vi "Write ECAT VARs.vi"(7 "R/W Case":T7, 8 "error in (no error)":errorcluster, 9 "Input FIFO buffer in":dbl[](array[numeric]), 10 "I/O Output Data in":T1 {"BD Refs"."Data Reference" format="%.0x"}, 11 "I/O Imput Vars in":T4[](array[typedef]) {"VS ref" format="%.0x"}) -> (0 "error out":errorcluster, 1 "Input FIFO buffer out":dbl[](array[numeric]), 2 "I/O Output Data out":T1 {"BD Refs"."Data Reference" format="%.0x"}, 3 "I/O Imput Vars out":T4[](array[typedef]) {"VS ref" format="%.0x"})   [LabVIEW 2015, in "Scan Engine Custom Device.lvlib"]
uses:
  Type Defs/RW Case.ctl
  Type Defs/Generic ECAT Slave IOV Cluster.ctl
  <vilib>/NI Veristand/Custom Device API/Custom Device Item Ref.ctl
  Type Defs/UDV Data Type.ctl
  Type Defs/Output Data.ctl
  <vilib>/NI Veristand/Custom Device API/Block Data Reference.ctl
  <vilib>/NI Veristand/Custom Device API/Data Reference.ctl
  <vilib>/NI Veristand/Custom Device API/Global Data Refs.vi
  Scan Engine Custom Device.lvlib
  <vilib>/NI Veristand/Custom Device API/Custom Device API.lvlib
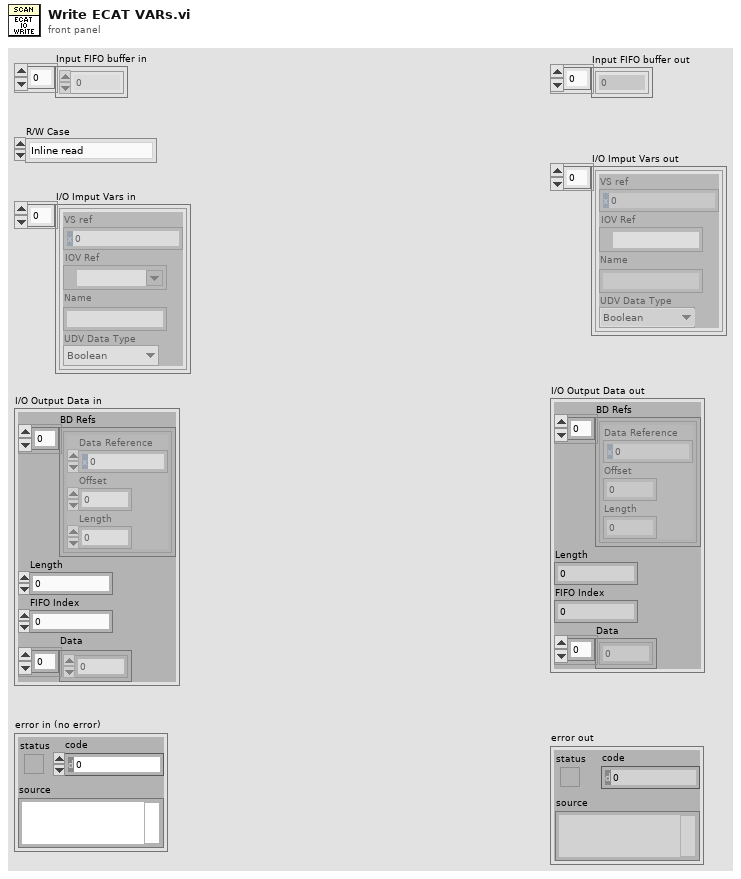
[diagram p1: front panel]
types:
  T1 = typedef "Scan Engine Custom Device.lvlib/Output Data.ctl" = cluster{"BD Refs":T2[], "Length":i32, "FIFO Index":i32, "Data":dbl[]}
  T2 = typedef "Custom Device API.lvlib/Block Data Reference.ctl" = cluster{"Data Reference":T3, "Offset":u64, "Length":u64}
  T3 = typedef "Custom Device API.lvlib/Data Reference.ctl" = i32
  T4 = typedef "Scan Engine Custom Device.lvlib/Generic ECAT Slave IOV Cluster.ctl" = cluster{"VS ref":T5, "IOV Ref":refnum<k21>, "Name":string, "UDV Data Type":T6}
  T5 = typedef "Custom Device API.lvlib/Custom Device Item Ref.ctl" = u64
  T6 = typedef "Scan Engine Custom Device.lvlib/UDV Data Type.ctl" = enum16{"Boolean", "Fixed Point", "Int8", "Int16", "Int32", "Int64", "U32 Bit Field", "UInt8", "UInt16", "UInt32", "UInt64", "Other"}
  T7 = typedef "Scan Engine Custom Device.lvlib/RW Case.ctl" = enum16{"Inline read", "Inline write", "Async - Inline loop read", "Async - Inline loop write", "Async loop (read/write)"}
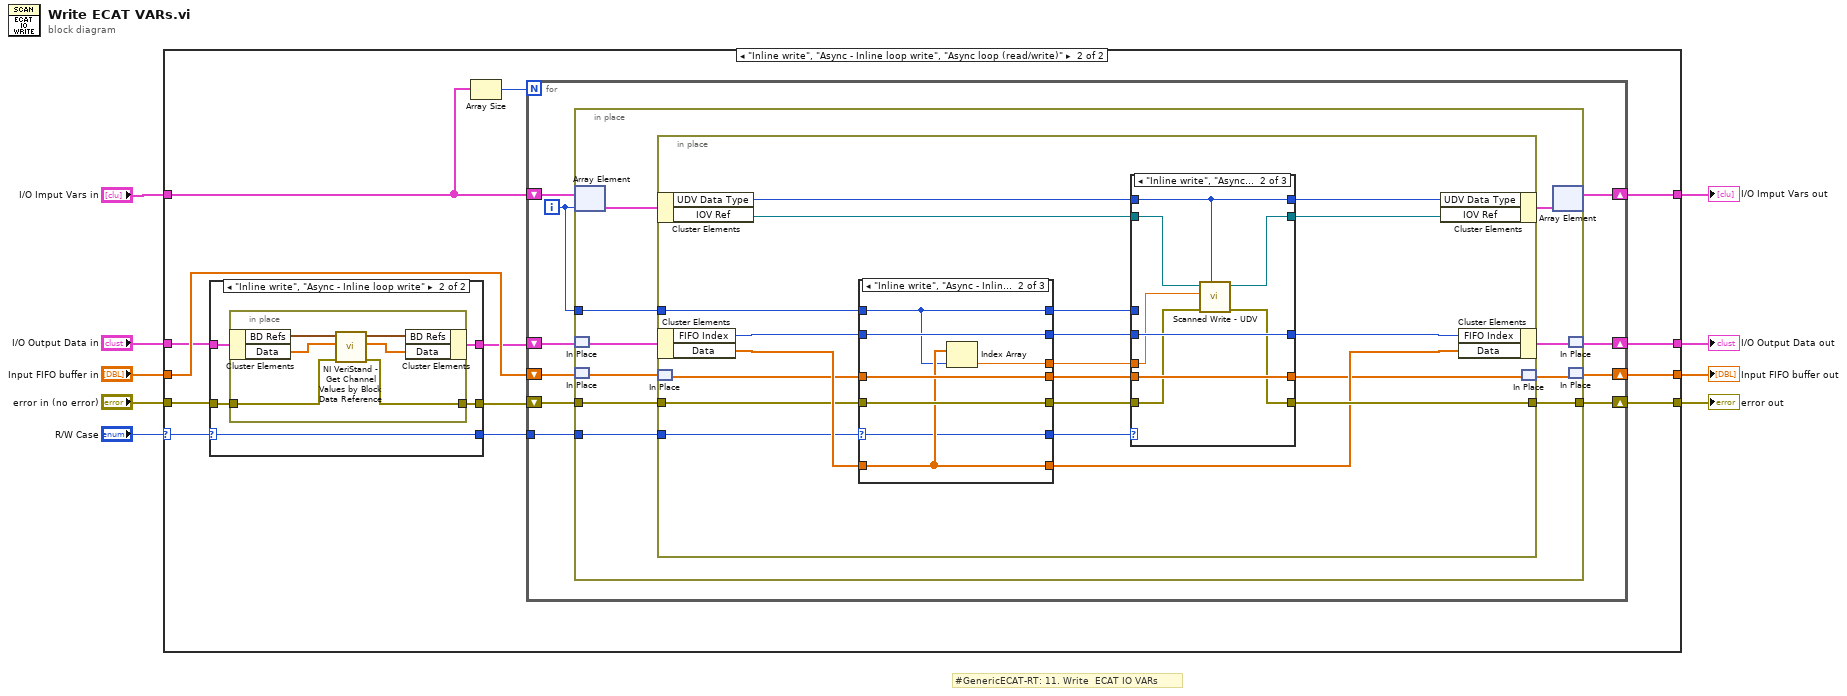
[diagram p0: block diagram]
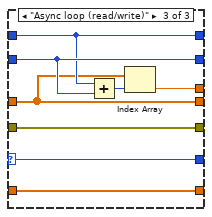
[diagram p5: hidden frame]
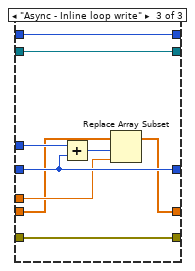
[diagram p7: hidden frame]
diagram:
  # "#GenericECAT-RT: 11. Write  ECAT IO VARs"
  n1 = case shown="\"Inline write\", \"Async - Inline loop write\", \"Async loop (read/write)\"" "R/W Case" {
    selector: "R/W Case" -> [_ w21]
    tunnel: [w11 w26] -> w9
    tunnel: "Input FIFO buffer in" -> [w11 w25]
    tunnel: [w12 w15] -> w2
    tunnel: [w13 w24] -> w3
    tunnel: "I/O Output Data in" -> [w12 w19]
    tunnel: "I/O Imput Vars in" -> [w13 w23]
    tunnel: [w10 w14] -> w7
    tunnel: "error in (no error)" -> [w10 w20]
    frame Default {
    }
    frame "Inline write", "Async - Inline loop write", "Async loop (read/write)" {
      n2 = case shown="\"Inline write\", \"Async - Inline loop write\"" w21 {
        selector: w21 -> [w27 w30]
        tunnel: w19 -> [w28 w34]
        tunnel: w20 -> [w29 w33]
        tunnel: [w29 w32] -> w17
        tunnel: [w28 w31] -> w18
        tunnel: [w27 w30] -> w16
        frame Default {
        }
        frame "Inline write", "Async - Inline loop write" {
          n3 = in-place {
            in-place-border: w33 -> [w36]
            in-place-border: [w35] -> w32
            n4 = in-place-cluster #1(w34) -> ("BD Refs"=w40:T2[], "Data"=w38:dbl[])
            n5 = call <vilib>:"NI VeriStand - Get Channel Values by Block Data Reference.vi"("error in (no error)"=w36, "Values Array in"=w38, "Block Data Ref"=w40) -> ("error out"=w35:errorcluster, "Values Array out"=w37:dbl[], "Block Data Ref dup"=w39:T2[])  [unwired: 6 in]
            n6 = in-place-cluster #1("BD Refs"=w39, "Data"=w37) -> (w31:T1)
          }
        }
      }
      n7 = Array Size(array=w23) -> (size(s)=w22:i32)
      n8 = for {
        N: w22 -> [_]
        shift-right: [w49] -> w24
        shift-left: w23 -> [w50]
        shift-right: [w41] -> w15
        shift-left: w18 -> [w44]
        shift-right: [w47] -> w26
        shift-left: w25 -> [w48]
        shift-right: [w45] -> w14
        shift-left: w17 -> [w46]
        tunnel: w16 -> [w43]
        i -> [w42]
        n9 = in-place {
          in-place-border: w46 -> [w57]
          in-place-border: [w51] -> w45
          in-place-border: w43 -> [w56]
          in-place-border: w42 -> [w55]
          n10 = in-place-array #2(w50, w42) -> (w60:T4)
          n11 = in-place-match #3(w44) -> (w59:T1)
          n12 = in-place-match #4(w48) -> (w58:dbl[])
          n13 = in-place {
            in-place-border: w57 -> [w74]
            in-place-border: w56 -> [w67]
            in-place-border: w55 -> [w75]
            in-place-border: [w71] -> w51
            n14 = in-place-cluster #5(w60) -> ("UDV Data Type"=w78:T6, "IOV Ref"=w77:refnum<k21>)
            n15 = in-place-cluster #6(w59) -> ("FIFO Index"=w80:i32, "Data"=w79:dbl[])
            n16 = in-place-match #7(w58) -> (w76:dbl[])
            n17 = case shown="\"Inline write\", \"Async - Inline loop write\"" w67 {
              selector: w67 -> [w83 w87 w94]
              tunnel: w75 -> [w81 w88 w96]
              tunnel: w80 -> [w86 w91 w99]
              tunnel: w76 -> [w84 w92 w95]
              tunnel: w74 -> [w82 w93 w101]
              tunnel: w79 -> [w85 w89 w100]
              tunnel: [w86 w91 w99] -> w63
              tunnel: [w85 w89 w100] -> w69
              tunnel: [w82 w93 w101] -> w65
              tunnel: [w84 w92 w95] -> w62
              tunnel: [w83 w87 w94] -> w66
              tunnel: [_ w90 w97] -> w61
              tunnel: [w81 w88 w96] -> w64
              frame Default {
              }
              frame "Inline write", "Async - Inline loop write" {
                n18 = Index Array(array=w89, index=w88) -> (element=w90:dbl)
              }
              frame "Async loop (read/write)" {
                n19 = Add(x=w96, y=w99) -> (x+y=w98:i32)
                n20 = Index Array(array=w95, index=w98) -> (element=w97:dbl)
              }
            }
            n21 = case shown="\"Inline write\", \"Async loop (read/write)\"" w66 {
              tunnel: w78 -> [w102 w110 w123]
              tunnel: w77 -> [w103 w112 w115]
              tunnel: w63 -> [w104 w113 w120]
              tunnel: w62 -> [w105 w114 w117]
              tunnel: [w105 w114 w116] -> w68
              tunnel: w64 -> [_ _ w121]
              tunnel: [w104 w113 w120] -> w70
              tunnel: [w103 w111 w115] -> w72
              tunnel: [w102 w110 w123] -> w73
              tunnel: w65 -> [w106 w108 w122]
              tunnel: [w106 w107 w122] -> w71
              tunnel: w61 -> [_ w109 w118]
              frame Default {
              }
              frame "Inline write", "Async loop (read/write)" {
                n22 = call "Scanned Write - UDV.vi"("UDV Data Type"=w110, "error in (no error)"=w108, "data in"=w109, "IOV ref in"=w112) -> ("error out"=w107:errorcluster, "IOV ref out"=w111:refnum<k21>)  [unwired: 6 in]
              }
              frame "Async - Inline loop write" {
                n23 = Add(x=w121, y=w120) -> (x+y=w119:i32)
                n24 = Replace Array Subset(array=w117, new element=w118, index=w119) -> (w116:dbl[])
              }
            }
            n25 = in-place-cluster #5("UDV Data Type"=w73, "IOV Ref"=w72) -> (w54:T4)
            n26 = in-place-cluster #6("FIFO Index"=w70, "Data"=w69) -> (w53:T1)
            n27 = in-place-match #7(w68) -> (w52:dbl[])
          }
          n28 = in-place-array #2(w54) -> (w49:T4[])  [unwired: 1 out]
          n29 = in-place-match #3(w53) -> (w41:T1)
          n30 = in-place-match #4(w52) -> (w47:dbl[])
        }
      }
    }
  }
  "Input FIFO buffer out" <- w9
  "error out" <- w7
  "I/O Imput Vars out" <- w3
  "I/O Output Data out" <- w2
